vi "AddConcession.vi"(8 "error in (no error)":errorcluster, 9 "Item to conceed":refnum<class "IDependencyItemRule.lvclass">, 11 "CDependencyItemRule in":refnum<class "CDependencyItemRule.lvclass">) -> (0 "error out":errorcluster, 3 "CDependencyItemRule out":refnum<class "CDependencyItemRule.lvclass">)   [LabVIEW 2020, in "LabVIEWContainers.lvlib" / "CDependencyItemRule.lvclass"]
uses:
  CDependencyItemRule.lvclass
  CDependencyItemRule.lvclass/CDependencyItemRule.ctl
  LabVIEWObjectInterfaces/IDependencyItemRule/IDependencyItemRule.lvclass
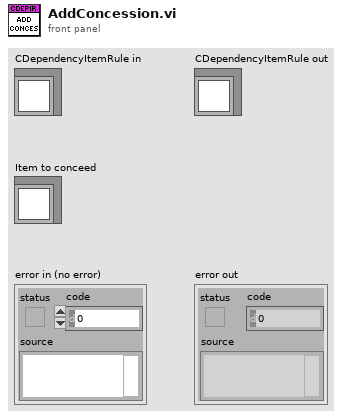
[diagram p1: front panel]
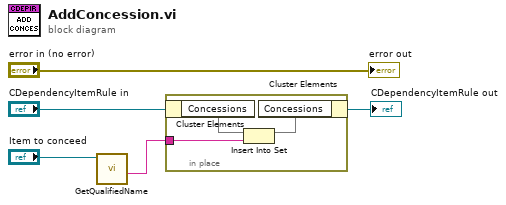
[diagram p0: block diagram]
diagram:
  n1 = call-dynamic "GetQualifiedName.vi"("ILabVIEWItem in"="Item to conceed") -> ("Qualified name"=w1:string)  [unwired: 8 in, 2 out]
  n2 = in-place {
    in-place-border: w1 -> [w6]
    n3 = in-place-cluster #1("CDependencyItemRule in") -> ("Concessions"=w8:set{string})
    n4 = Insert Into Set(10:w6, 11:w8) -> (3:w7:set{string})  [unwired: 1 out]
    n5 = in-place-cluster #1("Concessions"=w7) -> (→"CDependencyItemRule out":refnum<class "CDependencyItemRule.lvclass">)
  }
  "error out" <- "error in (no error)"
